vi "Tap Block Image (SubVI).vi"(5 "In Valid?":bool, 7 "Data In":u8) -> (4 "Ready for Input":bool)   [LabVIEW 2015]
uses:
  <vilib>/rvi/DataTransferAndStorage/Container/XNode/niFpgaContainer.xnode
  <vilib>/rvi/interface/RandomDataEmulation/nirviRandomDataFpgaReadWriteTemplate.vi
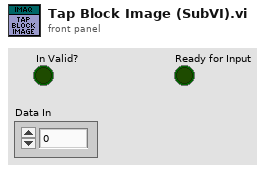
[diagram p1: front panel]
types:
  T1 = cluster{"[0]":u8, "[1]":u8, "[2]":u8, "[3]":u8, "[4]":u8, "[5]":u8, "[6]":u8, "[7]":u8}
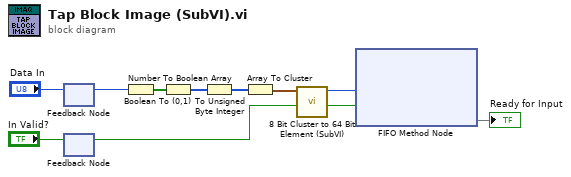
[diagram p0: block diagram]
diagram:
  n1 = feedback-in #1("Data In") -> ()
  n2 = feedback #1() -> (w2:u8)  [unwired: 1 in]
  n3 = feedback-in #2("In Valid?") -> ()
  n4 = feedback #2() -> (w3:bool)  [unwired: 1 in]
  n5 = Number To Boolean Array(number=w2) -> (Boolean array=w4:bool[])
  n6 = Boolean To (0,1)(Boolean=w4) -> (0, 1=w5:i16[])
  n7 = To Unsigned Byte Integer(number=w5) -> (unsigned 8bit integer=w7:u8[])
  n8 = Array To Cluster(array=w7) -> (cluster=w6:T1)
  n9 = call "8 Bit Cluster to 64 Bit Element (SubVI).vi"("Pixel Cluster"=w6) -> ("Pixel Data (64-Bit)"=w8:u64)  [unwired: 10 in]
  n10 = xnode ("FIFO Method Node")("Element"=w8, "Input Valid"=w3) -> ("Ready for Input"=→"Ready for Input")  [unwired: 1 in, 1 out]
